vi "Close MeasurementLink Session.vi"(8 "error in":errorcluster, 9 "close session behavior":T1, 10 "session in":variant, 11 "session factory in":refnum<class "Session Factory.lvclass">) -> (0 "error out":errorcluster)   [LabVIEW 2020, in "Keysight 34401A DMM Instrument.lvlib" / "Session Factory.lvclass"]
uses:
  Session Factory.lvclass
  <vilib>/MeasurementLink/MeasurementLink Instrument/ISession Factory/Initialize and Close Session Behavior.ctl
  <instrlib>/Agilent 34401/Public/Close.vi
  <instrlib>/Agilent 34401/Agilent 34401.lvlib
  <vilib>/MeasurementLink/MeasurementLink Instrument/ISession Factory/ISession Factory.lvclass
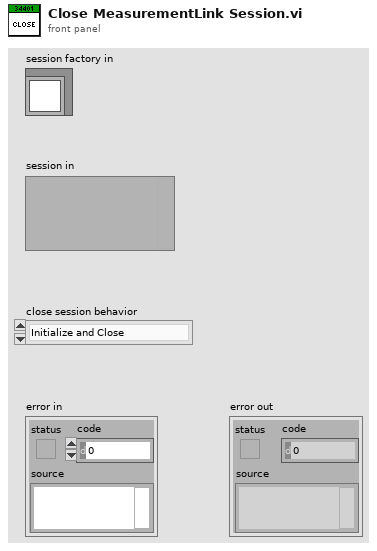
[diagram p1: front panel]
types:
  T1 = typedef "MeasurementLink Instrument.lvlib/ISession Factory.lvclass/Initialize and Close Session Behavior.ctl" = enum16{"Initialize and Close", "Attach and Detach", "Initialize and Detach", "Attach and Close"}
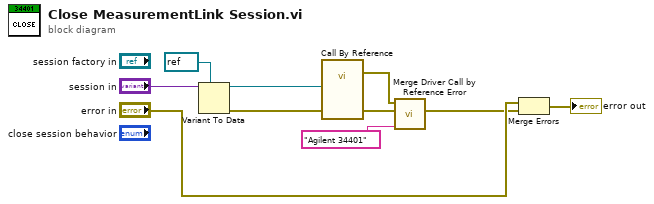
[diagram p0: block diagram]
diagram:
  n1 = Variant To Data(type=refnum<visa-resource-name> refnum ("VISA resource name out"), Variant="session in") -> (data=w6:refnum<visa-resource-name>, error out=w5:errorcluster)  [unwired: 1 in]
  n2 = call-by-ref "?"("error in (no error)"=w5, "VISA resource name"=w6) -> (error out=w3:errorcluster, 0:"error out"=w4:errorcluster)  [unwired: 11 in, 1 out]
  n3 = call <vilib>:"Merge Driver Call by Reference Error.vi"("driver name"="Agilent 34401", "called vi error"=w4, "call by ref error"=w3) -> ("error out"=w2:errorcluster)  [unwired: 8 in]
  n4 = Merge Errors("error in", w2) -> (→"error out":errorcluster)
